vi "麦格纳通讯test.vi"() -> ()   [LabVIEW 2014]
panel:
  out "写入成功 7":bool
  out "读取成功 14":bool
  out "写入成功 6":bool
  out "读取成功 13":bool
  out "写入成功 5":bool
  out "读取成功 12":bool
  out "写入成功 4":bool
  out "读取成功 11":bool
  out "写入成功 3":bool
  out "读取成功 10":bool
  out "写入成功 2":bool
  out "读取成功 9":bool
  out "读取成功 8":bool
  out "读取成功 7":bool
  out "读取成功 6":bool
  out "读取成功 5":bool
  out "读取成功 4":bool
  out "读取成功 3":bool
  out "读取成功 2":bool
  out "写入成功":bool
  out "读取成功":bool
  out "ST150 write":u32
  out "ST150 read":u32[](array[numeric])
  out "ST150":bool
  out "ST130 write":u32
  out "ST130 read":u32[](array[numeric])
  out "ST130":bool
  out "ST140 write":u32
  out "ST140 read":u32[](array[numeric])
  out "ST140":bool
  out "ST70 write":u32
  out "ST70 read":u32[](array[numeric])
  out "ST70":bool
  out "ST80 write":u32
  out "ST80 read":u32[](array[numeric])
  out "ST80":bool
  out "ST90 write":u32
  out "ST90 read":u32[](array[numeric])
  out "ST90":bool
  out "ST100 write":u32
  out "ST100 read":u32[](array[numeric])
  out "ST100":bool
  out "ST110 write":u32
  out "ST110 read":u32[](array[numeric])
  out "ST110":bool
  out "ST120 write":u32
  out "ST120 read":u32[](array[numeric])
  out "ST120":bool
  out "ST60 write":u32
  out "ST50 write":u32
  out "ST40 write":u32
  out "ST30 write":u32
  out "ST20 write":u32
  out "ST60 read":u32[](array[numeric])
  out "ST50 read":u32[](array[numeric])
  out "ST40 read":u32[](array[numeric])
  out "ST30 read":u32[](array[numeric])
  out "ST20 read":u32[](array[numeric])
  out "ST10 write":u32
  out "ST10 read":u32[](array[numeric])
  out "ST60":bool
  out "ST50":bool
  out "ST40":bool
  out "ST30":bool
  out "ST20":bool
  out "ST10":bool
  in  "停止":bool
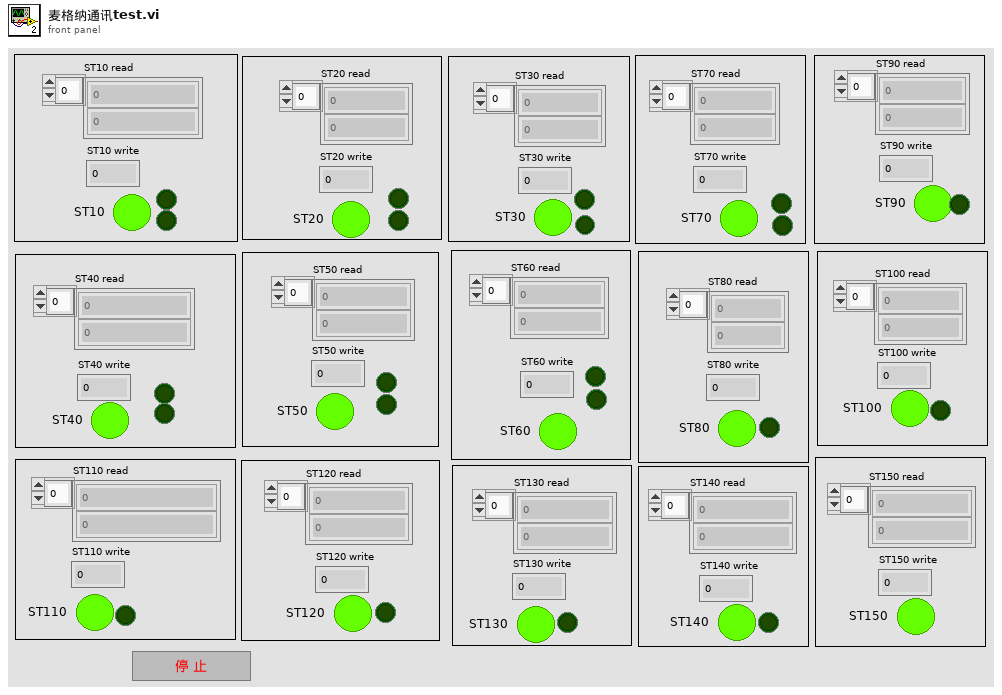
[diagram p1: front panel]
types:
  T1 = typedef "状态1.ctl" = enum16{"PLC通讯初始化", "读IO", "读DM", "写IO", "写DM", "-------------------", "仪表盘通讯初始化", "读数据", "保存曲线", "------------------", "错误"}
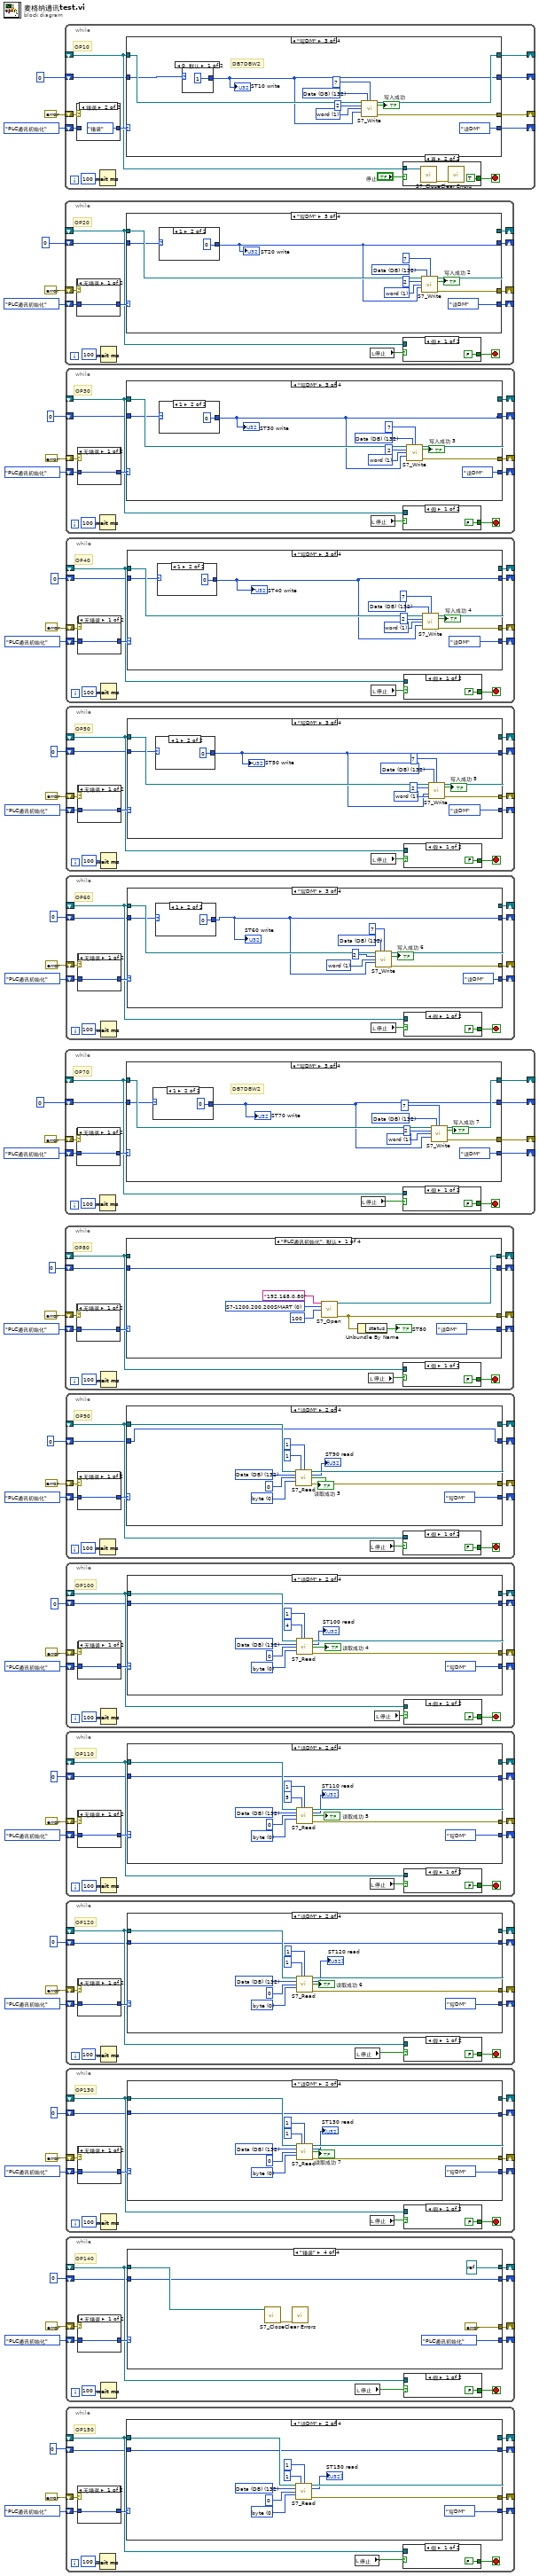
[diagram p0: block diagram]
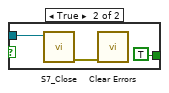
[diagram p2: hidden frame]
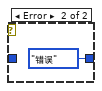
[diagram p3: hidden frame]
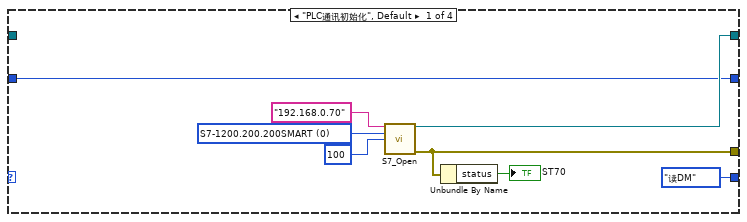
[diagram p4: hidden frame]
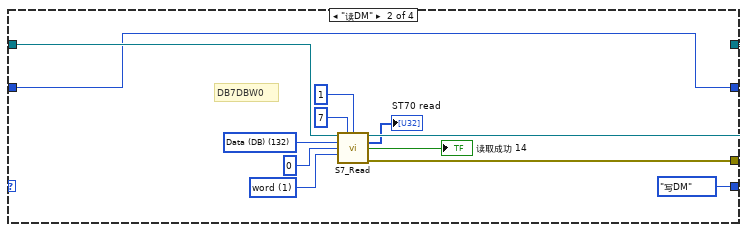
[diagram p5: hidden frame]
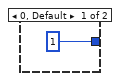
[diagram p6: hidden frame]
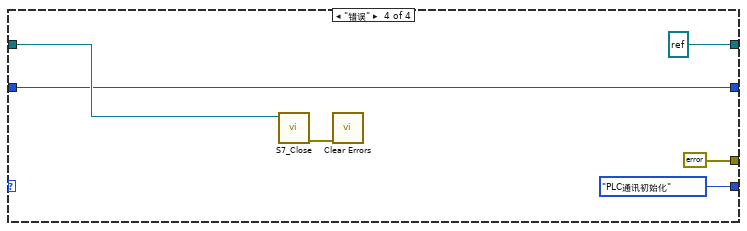
[diagram p7: hidden frame]
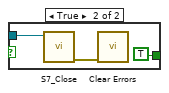
[diagram p8: hidden frame]
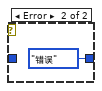
[diagram p9: hidden frame]
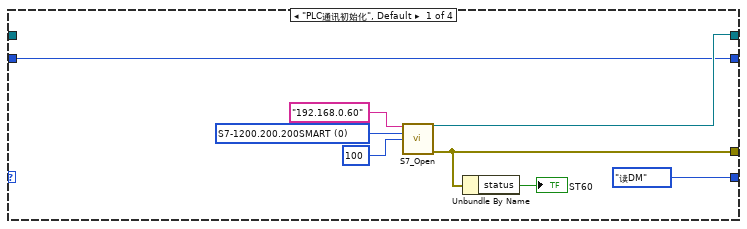
[diagram p10: hidden frame]
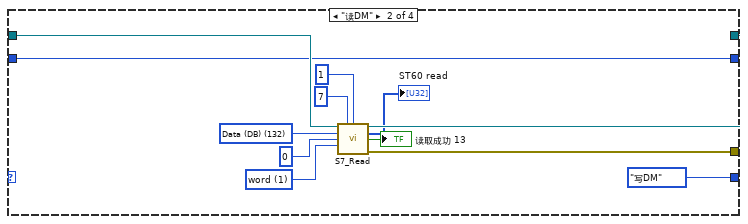
[diagram p11: hidden frame]
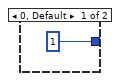
[diagram p12: hidden frame]
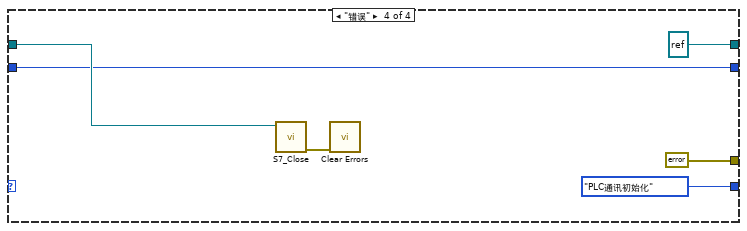
[diagram p13: hidden frame]
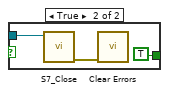
[diagram p14: hidden frame]
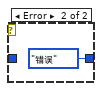
[diagram p15: hidden frame]
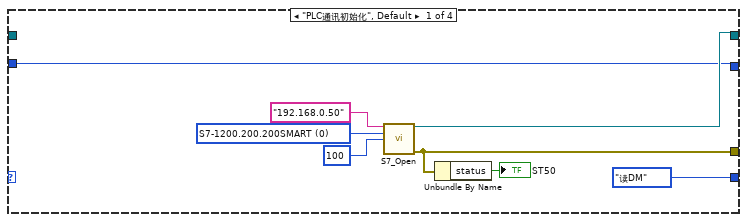
[diagram p16: hidden frame]
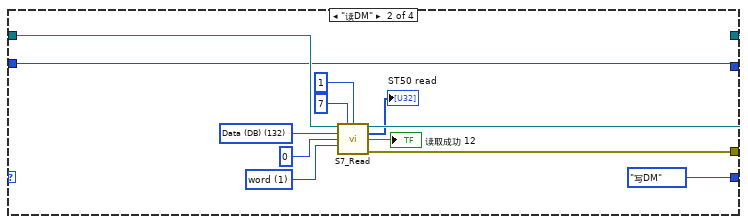
[diagram p17: hidden frame]
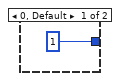
[diagram p18: hidden frame]
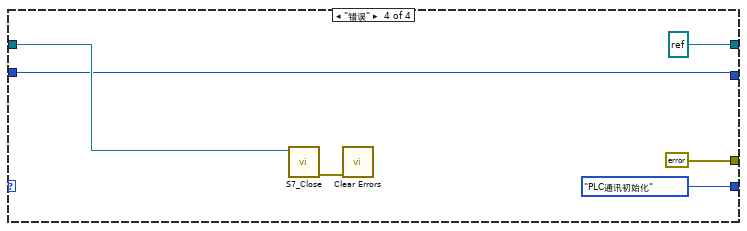
[diagram p19: hidden frame]
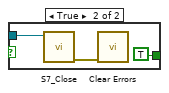
[diagram p20: hidden frame]
diagram:
  n1 = while {
    shift-right: [w51] -> _
    shift-left: 状态1."PLC通讯初始化" ("PLC状态") -> [w56]
    shift-right: [w53] -> _
    shift-left: errorcluster {"status"=FALSE, "code"=0, "source"=""} ("错误常量") -> [w57]
    shift-right: [w54] -> _
    shift-left: _ -> [w49]
    shift-right: [w46] -> _
    shift-left: u32 0 ("写入数据") -> [w47]
    stop <- w48 stop-if-true
    # "OP10"
    n2 = case shown="错误" w57 {
      tunnel: w56 -> [w62 _]
      tunnel: [w62 状态1."错误" ("PLC状态")] -> w55
      frame No Error {
      }
      frame Error {
      }
    }
    n3 = Wait (ms)(milliseconds to wait=u32 100 ("等待时间（毫秒）")) -> ()  [unwired: 1 out]
    n4 = case shown="\"写DM\"" w55 {
      tunnel: [w68 w78 w91 refnum<k5> refnum ("TCP")] -> w54
      tunnel: [w65 w77 w93 errorcluster {"status"=FALSE, "code"=0, "source"=""} ("error out")] -> w53
      tunnel: w49 -> [_ w79 w94 w102]
      tunnel: [状态1."读DM" ("PLC状态") 状态1."写DM" ("PLC状态") 状态1."读DM" ("PLC状态") 状态1."PLC通讯初始化" ("PLC状态")] -> w51
      tunnel: w47 -> [w66 w73 w86 w97]
      tunnel: [w66 w73 w85 w97] -> w46
      frame "PLC通讯初始化", Default {
        w70 = u8 0 items=["S7-1200.200.200SMART"=0, "S7-300"=2, "S7-400"=3] ("PLC 系列")
        n5 = call "S7_Open.vi"("IP 地址"="192.168.0.10", "PLC 系列"=w70, "超时（MS）"=100) -> ("TCP"=w68:refnum<k5>, "error out"=w65:errorcluster)  [unwired: 10 in, 1 out]
        n6 = Unbundle By Name(w65) -> ("status"=→"ST10":bool)
      }
      frame "读DM" {
        w80 = u16 1 items=["byte", "word", "Dword"] ("数据类型")
        w82 = u8 132 items=["I/O (P)"=128, "Input (I)"=129, "Output (Q)"=130, "Bit Memory (M)"=131, "Data (DB)"=132, "Instance Data (DI)"=133, "Local Data (L)"=134, "Predecessor Local Data (VL)"=135] ("寄存器类型")
        # "DB7DBW0"
        n7 = call "S7_Read.vi"("TCP"=w79, "DB #"=u16 7, "读取长度"=u16 1, "寄存器类型"=w82, "起始地址"=u32 0, "数据类型"=w80) -> ("TCP"=w78:refnum<k5>, "数据"=→"ST10 read":u32[], "读取成功"=→"读取成功":bool, "error out"=w77:errorcluster)  [unwired: 6 in]
      }
      frame "写DM" {
        w87 = u8 132 items=["I/O (P)"=128, "Input (I)"=129, "Output (Q)"=130, "Bit Memory (M)"=131, "Data (DB)"=132, "Instance Data (DI)"=133, "Local Data (L)"=134, "Predecessor Local Data (VL)"=135] ("寄存器类型")
        w89 = u16 1 items=["byte", "word", "Dword"] ("数据类型")
        # "DB7DBW2"
        n8 = case shown="0, 默认" w86 {
          tunnel: [u32 1 ("写入数据") u32 0 ("写入数据")] -> w85
          frame 0, Default {
          }
          frame 1 {
          }
        }
        "ST10 write" <- w85
        n9 = call "S7_Write.vi"("TCP"=w94, "寄存器类型"=w87, "DB #"=u16 7, "写入地址"=u32 2, "数据类型"=w89, "写入数据"=w85) -> ("TCP"=w91:refnum<k5>, "写入成功"=→"写入成功":bool, "error out"=w93:errorcluster)  [unwired: 7 in]
      }
      frame "错误" {
        n10 = call "S7_Close.vi"("TCP Connection Ref"=w102) -> ("error out"=w101:errorcluster)  [unwired: 10 in]
        n11 = call <vilib>:"Clear Errors.vi"("error in (no error)"=w101) -> ()  [unwired: 5 in, 2 out]
      }
    }
    n12 = case shown="真" "停止" {
      tunnel: w49 -> [_ w60]
      tunnel: [FALSE TRUE] -> w48
      frame False {
      }
      frame True {
        n13 = call "S7_Close.vi"("TCP Connection Ref"=w60) -> ("error out"=w61:errorcluster)  [unwired: 10 in]
        n14 = call <vilib>:"Clear Errors.vi"("error in (no error)"=w61) -> ()  [unwired: 5 in, 2 out]
      }
    }
  }
  n15 = while {
    shift-right: [w108] -> _
    shift-left: 状态1."PLC通讯初始化" ("PLC状态") -> [w113]
    shift-right: [w110] -> _
    shift-left: errorcluster {"status"=FALSE, "code"=0, "source"=""} ("错误常量") -> [w114]
    shift-right: [w111] -> _
    shift-left: _ -> [w107]
    shift-right: [w103] -> _
    shift-left: u32 0 ("写入数据") -> [w104]
    stop <- w106 stop-if-true
    # "OP20"
    n16 = case shown="无错误" w114 {
      tunnel: w113 -> [w119 _]
      tunnel: [w119 状态1."错误" ("PLC状态")] -> w112
      frame No Error {
      }
      frame Error {
      }
    }
    n17 = Wait (ms)(milliseconds to wait=u32 100 ("等待时间（毫秒）")) -> ()  [unwired: 1 out]
    n18 = case shown="\"写DM\"" w112 {
      tunnel: [w125 w135 w150 refnum<k5> refnum ("TCP")] -> w111
      tunnel: [w123 w134 w149 errorcluster {"status"=FALSE, "code"=0, "source"=""} ("error out")] -> w110
      tunnel: w107 -> [_ w136 w151 w159]
      tunnel: [状态1."读DM" ("PLC状态") 状态1."写DM" ("PLC状态") 状态1."读DM" ("PLC状态") 状态1."PLC通讯初始化" ("PLC状态")] -> w108
      tunnel: w104 -> [w121 w130 w143 w154]
      tunnel: [w121 w130 w142 w154] -> w103
      frame "PLC通讯初始化", Default {
        w127 = u8 0 items=["S7-1200.200.200SMART"=0, "S7-300"=2, "S7-400"=3] ("PLC 系列")
        n19 = call "S7_Open.vi"("IP 地址"="192.168.0.20", "PLC 系列"=w127, "超时（MS）"=100) -> ("TCP"=w125:refnum<k5>, "error out"=w123:errorcluster)  [unwired: 10 in, 1 out]
        n20 = Unbundle By Name(w123) -> ("status"=→"ST20":bool)
      }
      frame "读DM" {
        w137 = u16 1 items=["byte", "word", "Dword"] ("数据类型")
        w139 = u8 132 items=["I/O (P)"=128, "Input (I)"=129, "Output (Q)"=130, "Bit Memory (M)"=131, "Data (DB)"=132, "Instance Data (DI)"=133, "Local Data (L)"=134, "Predecessor Local Data (VL)"=135] ("寄存器类型")
        n21 = call "S7_Read.vi"("TCP"=w136, "DB #"=u16 7, "读取长度"=u16 1, "寄存器类型"=w139, "起始地址"=u32 0, "数据类型"=w137) -> ("TCP"=w135:refnum<k5>, "数据"=→"ST20 read":u32[], "读取成功"=→"读取成功 9":bool, "error out"=w134:errorcluster)  [unwired: 6 in]
      }
      frame "写DM" {
        w144 = u16 1 items=["byte", "word", "Dword"] ("数据类型")
        w146 = u8 132 items=["I/O (P)"=128, "Input (I)"=129, "Output (Q)"=130, "Bit Memory (M)"=131, "Data (DB)"=132, "Instance Data (DI)"=133, "Local Data (L)"=134, "Predecessor Local Data (VL)"=135] ("寄存器类型")
        n22 = case shown="1" w143 {
          tunnel: [u32 1 ("写入数据") u32 0 ("写入数据")] -> w142
          frame 0, Default {
          }
          frame 1 {
          }
        }
        "ST20 write" <- w142
        n23 = call "S7_Write.vi"("TCP"=w151, "寄存器类型"=w146, "DB #"=u16 7, "写入地址"=u32 2, "数据类型"=w144, "写入数据"=w142) -> ("TCP"=w150:refnum<k5>, "写入成功"=→"写入成功 2":bool, "error out"=w149:errorcluster)  [unwired: 7 in]
      }
      frame "错误" {
        n24 = call "S7_Close.vi"("TCP Connection Ref"=w159) -> ("error out"=w158:errorcluster)  [unwired: 10 in]
        n25 = call <vilib>:"Clear Errors.vi"("error in (no error)"=w158) -> ()  [unwired: 5 in, 2 out]
      }
    }
    n26 = local read "停止"() -> (w105:bool)
    n27 = case shown="假" w105 {
      tunnel: w107 -> [_ w117]
      tunnel: [FALSE TRUE] -> w106
      frame False {
      }
      frame True {
        n28 = call "S7_Close.vi"("TCP Connection Ref"=w117) -> ("error out"=w118:errorcluster)  [unwired: 10 in]
        n29 = call <vilib>:"Clear Errors.vi"("error in (no error)"=w118) -> ()  [unwired: 5 in, 2 out]
      }
    }
  }
  n30 = while {
    shift-right: [w165] -> _
    shift-left: 状态1."PLC通讯初始化" ("PLC状态") -> [w170]
    shift-right: [w167] -> _
    shift-left: errorcluster {"status"=FALSE, "code"=0, "source"=""} ("错误常量") -> [w171]
    shift-right: [w168] -> _
    shift-left: _ -> [w164]
    shift-right: [w161] -> _
    shift-left: u32 0 ("写入数据") -> [w162]
    stop <- w163 stop-if-true
    # "OP70"
    n31 = case shown="无错误" w171 {
      tunnel: w170 -> [w176 _]
      tunnel: [w176 状态1."错误" ("PLC状态")] -> w169
      frame No Error {
      }
      frame Error {
      }
    }
    n32 = Wait (ms)(milliseconds to wait=u32 100 ("等待时间（毫秒）")) -> ()  [unwired: 1 out]
    n33 = case shown="\"写DM\"" w169 {
      tunnel: [w182 w192 w205 refnum<k5> refnum ("TCP")] -> w168
      tunnel: [w180 w191 w207 errorcluster {"status"=FALSE, "code"=0, "source"=""} ("error out")] -> w167
      tunnel: w164 -> [_ w193 w208 w216]
      tunnel: [状态1."读DM" ("PLC状态") 状态1."写DM" ("PLC状态") 状态1."读DM" ("PLC状态") 状态1."PLC通讯初始化" ("PLC状态")] -> w165
      tunnel: w162 -> [w178 w187 w200 w211]
      tunnel: [w178 w187 w199 w211] -> w161
      frame "PLC通讯初始化", Default {
        w184 = u8 0 items=["S7-1200.200.200SMART"=0, "S7-300"=2, "S7-400"=3] ("PLC 系列")
        n34 = call "S7_Open.vi"("IP 地址"="192.168.0.70", "PLC 系列"=w184, "超时（MS）"=100) -> ("TCP"=w182:refnum<k5>, "error out"=w180:errorcluster)  [unwired: 10 in, 1 out]
        n35 = Unbundle By Name(w180) -> ("status"=→"ST70":bool)
      }
      frame "读DM" {
        w194 = u16 1 items=["byte", "word", "Dword"] ("数据类型")
        w196 = u8 132 items=["I/O (P)"=128, "Input (I)"=129, "Output (Q)"=130, "Bit Memory (M)"=131, "Data (DB)"=132, "Instance Data (DI)"=133, "Local Data (L)"=134, "Predecessor Local Data (VL)"=135] ("寄存器类型")
        # "DB7DBW0"
        n36 = call "S7_Read.vi"("TCP"=w193, "DB #"=u16 7, "读取长度"=u16 1, "寄存器类型"=w196, "起始地址"=u32 0, "数据类型"=w194) -> ("TCP"=w192:refnum<k5>, "数据"=→"ST70 read":u32[], "读取成功"=→"读取成功 14":bool, "error out"=w191:errorcluster)  [unwired: 6 in]
      }
      frame "写DM" {
        w201 = u8 132 items=["I/O (P)"=128, "Input (I)"=129, "Output (Q)"=130, "Bit Memory (M)"=131, "Data (DB)"=132, "Instance Data (DI)"=133, "Local Data (L)"=134, "Predecessor Local Data (VL)"=135] ("寄存器类型")
        w203 = u16 1 items=["byte", "word", "Dword"] ("数据类型")
        # "DB7DBW2"
        n37 = case shown="1" w200 {
          tunnel: [u32 1 ("写入数据") u32 0 ("写入数据")] -> w199
          frame 0, Default {
          }
          frame 1 {
          }
        }
        "ST70 write" <- w199
        n38 = call "S7_Write.vi"("TCP"=w208, "寄存器类型"=w201, "DB #"=u16 7, "写入地址"=u32 2, "数据类型"=w203, "写入数据"=w199) -> ("TCP"=w205:refnum<k5>, "写入成功"=→"写入成功 7":bool, "error out"=w207:errorcluster)  [unwired: 7 in]
      }
      frame "错误" {
        n39 = call "S7_Close.vi"("TCP Connection Ref"=w216) -> ("error out"=w215:errorcluster)  [unwired: 10 in]
        n40 = call <vilib>:"Clear Errors.vi"("error in (no error)"=w215) -> ()  [unwired: 5 in, 2 out]
      }
    }
    n41 = local read "停止"() -> (w160:bool)
    n42 = case shown="假" w160 {
      tunnel: w164 -> [_ w174]
      tunnel: [FALSE TRUE] -> w163
      frame False {
      }
      frame True {
        n43 = call "S7_Close.vi"("TCP Connection Ref"=w174) -> ("error out"=w175:errorcluster)  [unwired: 10 in]
        n44 = call <vilib>:"Clear Errors.vi"("error in (no error)"=w175) -> ()  [unwired: 5 in, 2 out]
      }
    }
  }
  n45 = while {
    shift-right: [w222] -> _
    shift-left: 状态1."PLC通讯初始化" ("PLC状态") -> [w227]
    shift-right: [w224] -> _
    shift-left: errorcluster {"status"=FALSE, "code"=0, "source"=""} ("错误常量") -> [w228]
    shift-right: [w225] -> _
    shift-left: _ -> [w221]
    shift-right: [w218] -> _
    shift-left: u32 0 ("写入数据") -> [w219]
    stop <- w220 stop-if-true
    # "OP80"
    n46 = case shown="无错误" w228 {
      tunnel: w227 -> [w233 _]
      tunnel: [w233 状态1."错误" ("PLC状态")] -> w226
      frame No Error {
      }
      frame Error {
      }
    }
    n47 = Wait (ms)(milliseconds to wait=u32 100 ("等待时间（毫秒）")) -> ()  [unwired: 1 out]
    n48 = case shown="\"PLC通讯初始化\", 默认" w226 {
      tunnel: [w239 w249 w259 refnum<k5> refnum ("TCP")] -> w225
      tunnel: [w237 w248 w258 errorcluster {"status"=FALSE, "code"=0, "source"=""} ("error out")] -> w224
      tunnel: w221 -> [_ w250 w260 w280]
      tunnel: [状态1."读DM" ("PLC状态") 状态1."写DM" ("PLC状态") 状态1."读DM" ("PLC状态") 状态1."PLC通讯初始化" ("PLC状态")] -> w222
      tunnel: w219 -> [w235 w244 w256 w275]
      tunnel: [w235 w244 w255 w275] -> w218
      frame "PLC通讯初始化", Default {
        w241 = u8 0 items=["S7-1200.200.200SMART"=0, "S7-300"=2, "S7-400"=3] ("PLC 系列")
        n49 = call "S7_Open.vi"("IP 地址"="192.168.0.80", "PLC 系列"=w241, "超时（MS）"=100) -> ("TCP"=w239:refnum<k5>, "error out"=w237:errorcluster)  [unwired: 10 in, 1 out]
        n50 = Unbundle By Name(w237) -> ("status"=→"ST80":bool)
      }
      frame "读DM" {
        w251 = u16 0 items=["byte", "word", "Dword"] ("数据类型")
        w253 = u8 132 items=["I/O (P)"=128, "Input (I)"=129, "Output (Q)"=130, "Bit Memory (M)"=131, "Data (DB)"=132, "Instance Data (DI)"=133, "Local Data (L)"=134, "Predecessor Local Data (VL)"=135] ("寄存器类型")
        n51 = call "S7_Read.vi"("TCP"=w250, "DB #"=u16 8, "读取长度"=u16 1, "寄存器类型"=w253, "起始地址"=u32 0, "数据类型"=w251) -> ("TCP"=w249:refnum<k5>, "数据"=→"ST80 read":u32[], "读取成功"=→"读取成功 2":bool, "error out"=w248:errorcluster)  [unwired: 6 in]
      }
      frame "写DM" {
        n52 = disable-structure shown="启用" {
          disable-tunnel: w260 -> [w269 w274]
          disable-tunnel: [w268 w274] -> w259
          disable-tunnel: [w267 errorcluster {"status"=FALSE, "code"=0, "source"=""} ("error out")] -> w258
          disable-tunnel: w256 -> [w262 w273]
          disable-tunnel: [w261 w273] -> w255
          frame Disabled {
            w263 = u16 1 items=["byte", "word", "Dword"] ("数据类型")
            w265 = u8 132 items=["I/O (P)"=128, "Input (I)"=129, "Output (Q)"=130, "Bit Memory (M)"=131, "Data (DB)"=132, "Instance Data (DI)"=133, "Local Data (L)"=134, "Predecessor Local Data (VL)"=135] ("寄存器类型")
            n53 = case shown="1" w262 {
              tunnel: [u32 1 ("写入数据") u32 0 ("写入数据")] -> w261
              frame 0, Default {
              }
              frame 1 {
              }
            }
            "ST80 write" <- w261
            n54 = call "S7_Write.vi"("TCP"=w269, "寄存器类型"=w265, "DB #"=u16 7, "写入地址"=u32 2, "数据类型"=w263, "写入数据"=w261) -> ("TCP"=w268:refnum<k5>, "error out"=w267:errorcluster)  [unwired: 7 in, 1 out]
          }
          frame Enabled {
          }
        }
      }
      frame "错误" {
        n55 = call "S7_Close.vi"("TCP Connection Ref"=w280) -> ("error out"=w279:errorcluster)  [unwired: 10 in]
        n56 = call <vilib>:"Clear Errors.vi"("error in (no error)"=w279) -> ()  [unwired: 5 in, 2 out]
      }
    }
    n57 = local read "停止"() -> (w217:bool)
    n58 = case shown="假" w217 {
      tunnel: w221 -> [_ w231]
      tunnel: [FALSE TRUE] -> w220
      frame False {
      }
      frame True {
        n59 = call "S7_Close.vi"("TCP Connection Ref"=w231) -> ("error out"=w232:errorcluster)  [unwired: 10 in]
        n60 = call <vilib>:"Clear Errors.vi"("error in (no error)"=w232) -> ()  [unwired: 5 in, 2 out]
      }
    }
  }
  n61 = while {
    shift-right: [w286] -> _
    shift-left: 状态1."PLC通讯初始化" ("PLC状态") -> [w291]
    shift-right: [w288] -> _
    shift-left: errorcluster {"status"=FALSE, "code"=0, "source"=""} ("错误常量") -> [w292]
    shift-right: [w289] -> _
    shift-left: _ -> [w285]
    shift-right: [w281] -> _
    shift-left: u32 0 ("写入数据") -> [w282]
    stop <- w284 stop-if-true
    # "OP30"
    n62 = case shown="无错误" w292 {
      tunnel: w291 -> [w297 _]
      tunnel: [w297 状态1."错误" ("PLC状态")] -> w290
      frame No Error {
      }
      frame Error {
      }
    }
    n63 = Wait (ms)(milliseconds to wait=u32 100 ("等待时间（毫秒）")) -> ()  [unwired: 1 out]
    n64 = case shown="\"写DM\"" w290 {
      tunnel: [w303 w313 w328 refnum<k5> refnum ("TCP")] -> w289
      tunnel: [w300 w312 w327 errorcluster {"status"=FALSE, "code"=0, "source"=""} ("error out")] -> w288
      tunnel: w285 -> [_ w314 w329 w337]
      tunnel: [状态1."读DM" ("PLC状态") 状态1."写DM" ("PLC状态") 状态1."读DM" ("PLC状态") 状态1."PLC通讯初始化" ("PLC状态")] -> w286
      tunnel: w282 -> [w299 w308 w325 w332]
      tunnel: [w299 w308 w320 w332] -> w281
      frame "PLC通讯初始化", Default {
        w305 = u8 0 items=["S7-1200.200.200SMART"=0, "S7-300"=2, "S7-400"=3] ("PLC 系列")
        n65 = call "S7_Open.vi"("IP 地址"="192.168.0.30", "PLC 系列"=w305, "超时（MS）"=100) -> ("TCP"=w303:refnum<k5>, "error out"=w300:errorcluster)  [unwired: 10 in, 1 out]
        n66 = Unbundle By Name(w300) -> ("status"=→"ST30":bool)
      }
      frame "读DM" {
        w315 = u16 1 items=["byte", "word", "Dword"] ("数据类型")
        w317 = u8 132 items=["I/O (P)"=128, "Input (I)"=129, "Output (Q)"=130, "Bit Memory (M)"=131, "Data (DB)"=132, "Instance Data (DI)"=133, "Local Data (L)"=134, "Predecessor Local Data (VL)"=135] ("寄存器类型")
        n67 = call "S7_Read.vi"("TCP"=w314, "DB #"=u16 7, "读取长度"=u16 1, "寄存器类型"=w317, "起始地址"=u32 0, "数据类型"=w315) -> ("TCP"=w313:refnum<k5>, "数据"=→"ST30 read":u32[], "读取成功"=→"读取成功 10":bool, "error out"=w312:errorcluster)  [unwired: 6 in]
      }
      frame "写DM" {
        w321 = u16 1 items=["byte", "word", "Dword"] ("数据类型")
        w324 = u8 132 items=["I/O (P)"=128, "Input (I)"=129, "Output (Q)"=130, "Bit Memory (M)"=131, "Data (DB)"=132, "Instance Data (DI)"=133, "Local Data (L)"=134, "Predecessor Local Data (VL)"=135] ("寄存器类型")
        n68 = case shown="1" w325 {
          tunnel: [u32 1 ("写入数据") u32 0 ("写入数据")] -> w320
          frame 0, Default {
          }
          frame 1 {
          }
        }
        "ST30 write" <- w320
        n69 = call "S7_Write.vi"("TCP"=w329, "寄存器类型"=w324, "DB #"=u16 7, "写入地址"=u32 2, "数据类型"=w321, "写入数据"=w320) -> ("TCP"=w328:refnum<k5>, "写入成功"=→"写入成功 3":bool, "error out"=w327:errorcluster)  [unwired: 7 in]
      }
      frame "错误" {
        n70 = call "S7_Close.vi"("TCP Connection Ref"=w337) -> ("error out"=w336:errorcluster)  [unwired: 10 in]
        n71 = call <vilib>:"Clear Errors.vi"("error in (no error)"=w336) -> ()  [unwired: 5 in, 2 out]
      }
    }
    n72 = local read "停止"() -> (w283:bool)
    n73 = case shown="假" w283 {
      tunnel: w285 -> [_ w295]
      tunnel: [FALSE TRUE] -> w284
      frame False {
      }
      frame True {
        n74 = call "S7_Close.vi"("TCP Connection Ref"=w295) -> ("error out"=w296:errorcluster)  [unwired: 10 in]
        n75 = call <vilib>:"Clear Errors.vi"("error in (no error)"=w296) -> ()  [unwired: 5 in, 2 out]
      }
    }
  }
  n76 = while {
    shift-right: [w343] -> _
    shift-left: 状态1."PLC通讯初始化" ("PLC状态") -> [w348]
    shift-right: [w345] -> _
    shift-left: errorcluster {"status"=FALSE, "code"=0, "source"=""} ("错误常量") -> [w349]
    shift-right: [w346] -> _
    shift-left: _ -> [w342]
    shift-right: [w339] -> _
    shift-left: u32 0 ("写入数据") -> [w340]
    stop <- w341 stop-if-true
    # "OP90"
    n77 = case shown="无错误" w349 {
      tunnel: w348 -> [w354 _]
      tunnel: [w354 状态1."错误" ("PLC状态")] -> w347
      frame No Error {
      }
      frame Error {
      }
    }
    n78 = Wait (ms)(milliseconds to wait=u32 100 ("等待时间（毫秒）")) -> ()  [unwired: 1 out]
    n79 = case shown="\"读DM\"" w347 {
      tunnel: [w360 w370 w380 refnum<k5> refnum ("TCP")] -> w346
      tunnel: [w357 w369 w379 errorcluster {"status"=FALSE, "code"=0, "source"=""} ("error out")] -> w345
      tunnel: w342 -> [_ w371 w381 w401]
      tunnel: [状态1."读DM" ("PLC状态") 状态1."写DM" ("PLC状态") 状态1."读DM" ("PLC状态") 状态1."PLC通讯初始化" ("PLC状态")] -> w343
      tunnel: w340 -> [w356 w365 w377 w396]
      tunnel: [w356 w365 w376 w396] -> w339
      frame "PLC通讯初始化", Default {
        w362 = u8 0 items=["S7-1200.200.200SMART"=0, "S7-300"=2, "S7-400"=3] ("PLC 系列")
        n80 = call "S7_Open.vi"("IP 地址"="192.168.0.90", "PLC 系列"=w362, "超时（MS）"=100) -> ("TCP"=w360:refnum<k5>, "error out"=w357:errorcluster)  [unwired: 10 in, 1 out]
        n81 = Unbundle By Name(w357) -> ("status"=→"ST90":bool)
      }
      frame "读DM" {
        w372 = u16 0 items=["byte", "word", "Dword"] ("数据类型")
        w374 = u8 132 items=["I/O (P)"=128, "Input (I)"=129, "Output (Q)"=130, "Bit Memory (M)"=131, "Data (DB)"=132, "Instance Data (DI)"=133, "Local Data (L)"=134, "Predecessor Local Data (VL)"=135] ("寄存器类型")
        n82 = call "S7_Read.vi"("TCP"=w371, "DB #"=u16 1, "读取长度"=u16 1, "寄存器类型"=w374, "起始地址"=u32 0, "数据类型"=w372) -> ("TCP"=w370:refnum<k5>, "数据"=→"ST90 read":u32[], "读取成功"=→"读取成功 3":bool, "error out"=w369:errorcluster)  [unwired: 6 in]
      }
      frame "写DM" {
        n83 = disable-structure shown="启用" {
          disable-tunnel: w381 -> [w390 w394]
          disable-tunnel: [w389 w394] -> w380
          disable-tunnel: [w388 errorcluster {"status"=FALSE, "code"=0, "source"=""} ("error out")] -> w379
          disable-tunnel: w377 -> [w387 w395]
          disable-tunnel: [w382 w395] -> w376
          frame Disabled {
            w383 = u16 1 items=["byte", "word", "Dword"] ("数据类型")
            w386 = u8 132 items=["I/O (P)"=128, "Input (I)"=129, "Output (Q)"=130, "Bit Memory (M)"=131, "Data (DB)"=132, "Instance Data (DI)"=133, "Local Data (L)"=134, "Predecessor Local Data (VL)"=135] ("寄存器类型")
            n84 = case shown="1" w387 {
              tunnel: [u32 1 ("写入数据") u32 0 ("写入数据")] -> w382
              frame 0, Default {
              }
              frame 1 {
              }
            }
            "ST90 write" <- w382
            n85 = call "S7_Write.vi"("TCP"=w390, "寄存器类型"=w386, "DB #"=u16 7, "写入地址"=u32 2, "数据类型"=w383, "写入数据"=w382) -> ("TCP"=w389:refnum<k5>, "error out"=w388:errorcluster)  [unwired: 7 in, 1 out]
          }
          frame Enabled {
          }
        }
      }
      frame "错误" {
        n86 = call "S7_Close.vi"("TCP Connection Ref"=w401) -> ("error out"=w400:errorcluster)  [unwired: 10 in]
        n87 = call <vilib>:"Clear Errors.vi"("error in (no error)"=w400) -> ()  [unwired: 5 in, 2 out]
      }
    }
    n88 = local read "停止"() -> (w338:bool)
    n89 = case shown="假" w338 {
      tunnel: w342 -> [_ w352]
      tunnel: [FALSE TRUE] -> w341
      frame False {
      }
      frame True {
        n90 = call "S7_Close.vi"("TCP Connection Ref"=w352) -> ("error out"=w353:errorcluster)  [unwired: 10 in]
        n91 = call <vilib>:"Clear Errors.vi"("error in (no error)"=w353) -> ()  [unwired: 5 in, 2 out]
      }
    }
  }
  n92 = while {
    shift-right: [w407] -> _
    shift-left: 状态1."PLC通讯初始化" ("PLC状态") -> [w412]
    shift-right: [w409] -> _
    shift-left: errorcluster {"status"=FALSE, "code"=0, "source"=""} ("错误常量") -> [w413]
    shift-right: [w410] -> _
    shift-left: _ -> [w406]
    shift-right: [w403] -> _
    shift-left: u32 0 ("写入数据") -> [w404]
    stop <- w405 stop-if-true
    # "OP150"
    n93 = case shown="无错误" w413 {
      tunnel: w412 -> [w418 _]
      tunnel: [w418 状态1."错误" ("PLC状态")] -> w411
      frame No Error {
      }
      frame Error {
      }
    }
    n94 = Wait (ms)(milliseconds to wait=u32 100 ("等待时间（毫秒）")) -> ()  [unwired: 1 out]
    n95 = case shown="\"读DM\"" w411 {
      tunnel: [w424 w433 w443 refnum<k5> refnum ("TCP")] -> w410
      tunnel: [w421 w432 w442 errorcluster {"status"=FALSE, "code"=0, "source"=""} ("error out")] -> w409
      tunnel: w406 -> [_ w434 w444 w464]
      tunnel: [状态1."读DM" ("PLC状态") 状态1."写DM" ("PLC状态") 状态1."读DM" ("PLC状态") 状态1."PLC通讯初始化" ("PLC状态")] -> w407
      tunnel: w404 -> [w420 w428 w440 w459]
      tunnel: [w420 w428 w439 w459] -> w403
      frame "PLC通讯初始化", Default {
        w426 = u8 0 items=["S7-1200.200.200SMART"=0, "S7-300"=2, "S7-400"=3] ("PLC 系列")
        n96 = call "S7_Open.vi"("IP 地址"="192.168.0.150", "PLC 系列"=w426, "超时（MS）"=100) -> ("TCP"=w424:refnum<k5>, "error out"=w421:errorcluster)  [unwired: 10 in, 1 out]
        n97 = Unbundle By Name(w421) -> ("status"=→"ST150":bool)
      }
      frame "读DM" {
        w435 = u16 0 items=["byte", "word", "Dword"] ("数据类型")
        w437 = u8 132 items=["I/O (P)"=128, "Input (I)"=129, "Output (Q)"=130, "Bit Memory (M)"=131, "Data (DB)"=132, "Instance Data (DI)"=133, "Local Data (L)"=134, "Predecessor Local Data (VL)"=135] ("寄存器类型")
        n98 = call "S7_Read.vi"("TCP"=w434, "DB #"=u16 1, "读取长度"=u16 1, "寄存器类型"=w437, "起始地址"=u32 0, "数据类型"=w435) -> ("TCP"=w433:refnum<k5>, "数据"=→"ST150 read":u32[], "error out"=w432:errorcluster)  [unwired: 6 in, 1 out]
      }
      frame "写DM" {
        n99 = disable-structure shown="启用" {
          disable-tunnel: w444 -> [w453 w457]
          disable-tunnel: [w452 w457] -> w443
          disable-tunnel: [w451 errorcluster {"status"=FALSE, "code"=0, "source"=""} ("error out")] -> w442
          disable-tunnel: w440 -> [w450 w458]
          disable-tunnel: [w445 w458] -> w439
          frame Disabled {
            w446 = u16 1 items=["byte", "word", "Dword"] ("数据类型")
            w448 = u8 132 items=["I/O (P)"=128, "Input (I)"=129, "Output (Q)"=130, "Bit Memory (M)"=131, "Data (DB)"=132, "Instance Data (DI)"=133, "Local Data (L)"=134, "Predecessor Local Data (VL)"=135] ("寄存器类型")
            n100 = case shown="1" w450 {
              tunnel: [u32 1 ("写入数据") u32 0 ("写入数据")] -> w445
              frame 0, Default {
              }
              frame 1 {
              }
            }
            "ST150 write" <- w445
            n101 = call "S7_Write.vi"("TCP"=w453, "寄存器类型"=w448, "DB #"=u16 7, "写入地址"=u32 2, "数据类型"=w446, "写入数据"=w445) -> ("TCP"=w452:refnum<k5>, "error out"=w451:errorcluster)  [unwired: 7 in, 1 out]
          }
          frame Enabled {
          }
        }
      }
      frame "错误" {
        n102 = call "S7_Close.vi"("TCP Connection Ref"=w464) -> ("error out"=w463:errorcluster)  [unwired: 10 in]
        n103 = call <vilib>:"Clear Errors.vi"("error in (no error)"=w463) -> ()  [unwired: 5 in, 2 out]
      }
    }
    n104 = local read "停止"() -> (w402:bool)
    n105 = case shown="假" w402 {
      tunnel: w406 -> [_ w416]
      tunnel: [FALSE TRUE] -> w405
      frame False {
      }
      frame True {
        n106 = call "S7_Close.vi"("TCP Connection Ref"=w416) -> ("error out"=w417:errorcluster)  [unwired: 10 in]
        n107 = call <vilib>:"Clear Errors.vi"("error in (no error)"=w417) -> ()  [unwired: 5 in, 2 out]
      }
    }
  }
  n108 = while {
    shift-right: [w470] -> _
    shift-left: 状态1."PLC通讯初始化" ("PLC状态") -> [w475]
    shift-right: [w472] -> _
    shift-left: errorcluster {"status"=FALSE, "code"=0, "source"=""} ("错误常量") -> [w476]
    shift-right: [w473] -> _
    shift-left: _ -> [w469]
    shift-right: [w465] -> _
    shift-left: u32 0 ("写入数据") -> [w466]
    stop <- w468 stop-if-true
    # "OP40"
    n109 = case shown="无错误" w476 {
      tunnel: w475 -> [w481 _]
      tunnel: [w481 状态1."错误" ("PLC状态")] -> w474
      frame No Error {
      }
      frame Error {
      }
    }
    n110 = Wait (ms)(milliseconds to wait=u32 100 ("等待时间（毫秒）")) -> ()  [unwired: 1 out]
    n111 = case shown="\"写DM\"" w474 {
      tunnel: [w487 w497 w512 refnum<k5> refnum ("TCP")] -> w473
      tunnel: [w484 w496 w511 errorcluster {"status"=FALSE, "code"=0, "source"=""} ("error out")] -> w472
      tunnel: w469 -> [_ w498 w513 w521]
      tunnel: [状态1."读DM" ("PLC状态") 状态1."写DM" ("PLC状态") 状态1."读DM" ("PLC状态") 状态1."PLC通讯初始化" ("PLC状态")] -> w470
      tunnel: w466 -> [w483 w492 w509 w516]
      tunnel: [w483 w492 w504 w516] -> w465
      frame "PLC通讯初始化", Default {
        w489 = u8 0 items=["S7-1200.200.200SMART"=0, "S7-300"=2, "S7-400"=3] ("PLC 系列")
        n112 = call "S7_Open.vi"("IP 地址"="192.168.0.40", "PLC 系列"=w489, "超时（MS）"=100) -> ("TCP"=w487:refnum<k5>, "error out"=w484:errorcluster)  [unwired: 10 in, 1 out]
        n113 = Unbundle By Name(w484) -> ("status"=→"ST40":bool)
      }
      frame "读DM" {
        w499 = u16 1 items=["byte", "word", "Dword"] ("数据类型")
        w501 = u8 132 items=["I/O (P)"=128, "Input (I)"=129, "Output (Q)"=130, "Bit Memory (M)"=131, "Data (DB)"=132, "Instance Data (DI)"=133, "Local Data (L)"=134, "Predecessor Local Data (VL)"=135] ("寄存器类型")
        n114 = call "S7_Read.vi"("TCP"=w498, "DB #"=u16 7, "读取长度"=u16 1, "寄存器类型"=w501, "起始地址"=u32 0, "数据类型"=w499) -> ("TCP"=w497:refnum<k5>, "数据"=→"ST40 read":u32[], "读取成功"=→"读取成功 11":bool, "error out"=w496:errorcluster)  [unwired: 6 in]
      }
      frame "写DM" {
        w505 = u16 1 items=["byte", "word", "Dword"] ("数据类型")
        w507 = u8 132 items=["I/O (P)"=128, "Input (I)"=129, "Output (Q)"=130, "Bit Memory (M)"=131, "Data (DB)"=132, "Instance Data (DI)"=133, "Local Data (L)"=134, "Predecessor Local Data (VL)"=135] ("寄存器类型")
        n115 = case shown="1" w509 {
          tunnel: [u32 1 ("写入数据") u32 0 ("写入数据")] -> w504
          frame 0, Default {
          }
          frame 1 {
          }
        }
        "ST40 write" <- w504
        n116 = call "S7_Write.vi"("TCP"=w513, "寄存器类型"=w507, "DB #"=u16 7, "写入地址"=u32 2, "数据类型"=w505, "写入数据"=w504) -> ("TCP"=w512:refnum<k5>, "写入成功"=→"写入成功 4":bool, "error out"=w511:errorcluster)  [unwired: 7 in]
      }
      frame "错误" {
        n117 = call "S7_Close.vi"("TCP Connection Ref"=w521) -> ("error out"=w520:errorcluster)  [unwired: 10 in]
        n118 = call <vilib>:"Clear Errors.vi"("error in (no error)"=w520) -> ()  [unwired: 5 in, 2 out]
      }
    }
    n119 = local read "停止"() -> (w467:bool)
    n120 = case shown="假" w467 {
      tunnel: w469 -> [_ w479]
      tunnel: [FALSE TRUE] -> w468
      frame False {
      }
      frame True {
        n121 = call "S7_Close.vi"("TCP Connection Ref"=w479) -> ("error out"=w480:errorcluster)  [unwired: 10 in]
        n122 = call <vilib>:"Clear Errors.vi"("error in (no error)"=w480) -> ()  [unwired: 5 in, 2 out]
      }
    }
  }
  n123 = while {
    shift-right: [w527] -> _
    shift-left: 状态1."PLC通讯初始化" ("PLC状态") -> [w532]
    shift-right: [w529] -> _
    shift-left: errorcluster {"status"=FALSE, "code"=0, "source"=""} ("错误常量") -> [w533]
    shift-right: [w530] -> _
    shift-left: _ -> [w526]
    shift-right: [w522] -> _
    shift-left: u32 0 ("写入数据") -> [w523]
    stop <- w525 stop-if-true
    # "OP50"
    n124 = case shown="无错误" w533 {
      tunnel: w532 -> [w538 _]
      tunnel: [w538 状态1."错误" ("PLC状态")] -> w531
      frame No Error {
      }
      frame Error {
      }
    }
    n125 = Wait (ms)(milliseconds to wait=u32 100 ("等待时间（毫秒）")) -> ()  [unwired: 1 out]
    n126 = case shown="\"写DM\"" w531 {
      tunnel: [w544 w554 w569 refnum<k5> refnum ("TCP")] -> w530
      tunnel: [w541 w553 w568 errorcluster {"status"=FALSE, "code"=0, "source"=""} ("error out")] -> w529
      tunnel: w526 -> [_ w555 w570 w578]
      tunnel: [状态1."读DM" ("PLC状态") 状态1."写DM" ("PLC状态") 状态1."读DM" ("PLC状态") 状态1."PLC通讯初始化" ("PLC状态")] -> w527
      tunnel: w523 -> [w540 w549 w566 w573]
      tunnel: [w540 w549 w561 w573] -> w522
      frame "PLC通讯初始化", Default {
        w546 = u8 0 items=["S7-1200.200.200SMART"=0, "S7-300"=2, "S7-400"=3] ("PLC 系列")
        n127 = call "S7_Open.vi"("IP 地址"="192.168.0.50", "PLC 系列"=w546, "超时（MS）"=100) -> ("TCP"=w544:refnum<k5>, "error out"=w541:errorcluster)  [unwired: 10 in, 1 out]
        n128 = Unbundle By Name(w541) -> ("status"=→"ST50":bool)
      }
      frame "读DM" {
        w556 = u16 1 items=["byte", "word", "Dword"] ("数据类型")
        w558 = u8 132 items=["I/O (P)"=128, "Input (I)"=129, "Output (Q)"=130, "Bit Memory (M)"=131, "Data (DB)"=132, "Instance Data (DI)"=133, "Local Data (L)"=134, "Predecessor Local Data (VL)"=135] ("寄存器类型")
        n129 = call "S7_Read.vi"("TCP"=w555, "DB #"=u16 7, "读取长度"=u16 1, "寄存器类型"=w558, "起始地址"=u32 0, "数据类型"=w556) -> ("TCP"=w554:refnum<k5>, "数据"=→"ST50 read":u32[], "读取成功"=→"读取成功 12":bool, "error out"=w553:errorcluster)  [unwired: 6 in]
      }
      frame "写DM" {
        w562 = u16 1 items=["byte", "word", "Dword"] ("数据类型")
        w564 = u8 132 items=["I/O (P)"=128, "Input (I)"=129, "Output (Q)"=130, "Bit Memory (M)"=131, "Data (DB)"=132, "Instance Data (DI)"=133, "Local Data (L)"=134, "Predecessor Local Data (VL)"=135] ("寄存器类型")
        n130 = case shown="1" w566 {
          tunnel: [u32 1 ("写入数据") u32 0 ("写入数据")] -> w561
          frame 0, Default {
          }
          frame 1 {
          }
        }
        "ST50 write" <- w561
        n131 = call "S7_Write.vi"("TCP"=w570, "寄存器类型"=w564, "DB #"=u16 7, "写入地址"=u32 2, "数据类型"=w562, "写入数据"=w561) -> ("TCP"=w569:refnum<k5>, "写入成功"=→"写入成功 5":bool, "error out"=w568:errorcluster)  [unwired: 7 in]
      }
      frame "错误" {
        n132 = call "S7_Close.vi"("TCP Connection Ref"=w578) -> ("error out"=w577:errorcluster)  [unwired: 10 in]
        n133 = call <vilib>:"Clear Errors.vi"("error in (no error)"=w577) -> ()  [unwired: 5 in, 2 out]
      }
    }
    n134 = local read "停止"() -> (w524:bool)
    n135 = case shown="假" w524 {
      tunnel: w526 -> [_ w536]
      tunnel: [FALSE TRUE] -> w525
      frame False {
      }
      frame True {
        n136 = call "S7_Close.vi"("TCP Connection Ref"=w536) -> ("error out"=w537:errorcluster)  [unwired: 10 in]
        n137 = call <vilib>:"Clear Errors.vi"("error in (no error)"=w537) -> ()  [unwired: 5 in, 2 out]
      }
    }
  }
  n138 = while {
    shift-right: [w584] -> _
    shift-left: 状态1."PLC通讯初始化" ("PLC状态") -> [w589]
    shift-right: [w586] -> _
    shift-left: errorcluster {"status"=FALSE, "code"=0, "source"=""} ("错误常量") -> [w590]
    shift-right: [w587] -> _
    shift-left: _ -> [w583]
    shift-right: [w579] -> _
    shift-left: u32 0 ("写入数据") -> [w580]
    stop <- w582 stop-if-true
    # "OP60"
    n139 = case shown="无错误" w590 {
      tunnel: w589 -> [w595 _]
      tunnel: [w595 状态1."错误" ("PLC状态")] -> w588
      frame No Error {
      }
      frame Error {
      }
    }
    n140 = Wait (ms)(milliseconds to wait=u32 100 ("等待时间（毫秒）")) -> ()  [unwired: 1 out]
    n141 = case shown="\"写DM\"" w588 {
      tunnel: [w601 w611 w626 refnum<k5> refnum ("TCP")] -> w587
      tunnel: [w598 w610 w625 errorcluster {"status"=FALSE, "code"=0, "source"=""} ("error out")] -> w586
      tunnel: w583 -> [_ w612 w627 w635]
      tunnel: [状态1."读DM" ("PLC状态") 状态1."写DM" ("PLC状态") 状态1."读DM" ("PLC状态") 状态1."PLC通讯初始化" ("PLC状态")] -> w584
      tunnel: w580 -> [w597 w606 w623 w630]
      tunnel: [w597 w606 w618 w630] -> w579
      frame "PLC通讯初始化", Default {
        w603 = u8 0 items=["S7-1200.200.200SMART"=0, "S7-300"=2, "S7-400"=3] ("PLC 系列")
        n142 = call "S7_Open.vi"("IP 地址"="192.168.0.60", "PLC 系列"=w603, "超时（MS）"=100) -> ("TCP"=w601:refnum<k5>, "error out"=w598:errorcluster)  [unwired: 10 in, 1 out]
        n143 = Unbundle By Name(w598) -> ("status"=→"ST60":bool)
      }
      frame "读DM" {
        w613 = u16 1 items=["byte", "word", "Dword"] ("数据类型")
        w615 = u8 132 items=["I/O (P)"=128, "Input (I)"=129, "Output (Q)"=130, "Bit Memory (M)"=131, "Data (DB)"=132, "Instance Data (DI)"=133, "Local Data (L)"=134, "Predecessor Local Data (VL)"=135] ("寄存器类型")
        n144 = call "S7_Read.vi"("TCP"=w612, "DB #"=u16 7, "读取长度"=u16 1, "寄存器类型"=w615, "起始地址"=u32 0, "数据类型"=w613) -> ("TCP"=w611:refnum<k5>, "数据"=→"ST60 read":u32[], "读取成功"=→"读取成功 13":bool, "error out"=w610:errorcluster)  [unwired: 6 in]
      }
      frame "写DM" {
        w619 = u16 1 items=["byte", "word", "Dword"] ("数据类型")
        w621 = u8 132 items=["I/O (P)"=128, "Input (I)"=129, "Output (Q)"=130, "Bit Memory (M)"=131, "Data (DB)"=132, "Instance Data (DI)"=133, "Local Data (L)"=134, "Predecessor Local Data (VL)"=135] ("寄存器类型")
        n145 = case shown="1" w623 {
          tunnel: [u32 1 ("写入数据") u32 0 ("写入数据")] -> w618
          frame 0, Default {
          }
          frame 1 {
          }
        }
        "ST60 write" <- w618
        n146 = call "S7_Write.vi"("TCP"=w627, "寄存器类型"=w621, "DB #"=u16 7, "写入地址"=u32 2, "数据类型"=w619, "写入数据"=w618) -> ("TCP"=w626:refnum<k5>, "写入成功"=→"写入成功 6":bool, "error out"=w625:errorcluster)  [unwired: 7 in]
      }
      frame "错误" {
        n147 = call "S7_Close.vi"("TCP Connection Ref"=w635) -> ("error out"=w634:errorcluster)  [unwired: 10 in]
        n148 = call <vilib>:"Clear Errors.vi"("error in (no error)"=w634) -> ()  [unwired: 5 in, 2 out]
      }
    }
    n149 = local read "停止"() -> (w581:bool)
    n150 = case shown="假" w581 {
      tunnel: w583 -> [_ w593]
      tunnel: [FALSE TRUE] -> w582
      frame False {
      }
      frame True {
        n151 = call "S7_Close.vi"("TCP Connection Ref"=w593) -> ("error out"=w594:errorcluster)  [unwired: 10 in]
        n152 = call <vilib>:"Clear Errors.vi"("error in (no error)"=w594) -> ()  [unwired: 5 in, 2 out]
      }
    }
  }
  n153 = while {
    shift-right: [w641] -> _
    shift-left: 状态1."PLC通讯初始化" ("PLC状态") -> [w646]
    shift-right: [w643] -> _
    shift-left: errorcluster {"status"=FALSE, "code"=0, "source"=""} ("错误常量") -> [w647]
    shift-right: [w644] -> _
    shift-left: _ -> [w640]
    shift-right: [w637] -> _
    shift-left: u32 0 ("写入数据") -> [w638]
    stop <- w639 stop-if-true
    # "OP100"
    n154 = case shown="无错误" w647 {
      tunnel: w646 -> [w652 _]
      tunnel: [w652 状态1."错误" ("PLC状态")] -> w645
      frame No Error {
      }
      frame Error {
      }
    }
    n155 = Wait (ms)(milliseconds to wait=u32 100 ("等待时间（毫秒）")) -> ()  [unwired: 1 out]
    n156 = case shown="\"读DM\"" w645 {
      tunnel: [w658 w668 w678 refnum<k5> refnum ("TCP")] -> w644
      tunnel: [w655 w667 w677 errorcluster {"status"=FALSE, "code"=0, "source"=""} ("error out")] -> w643
      tunnel: w640 -> [_ w669 w679 w699]
      tunnel: [状态1."读DM" ("PLC状态") 状态1."写DM" ("PLC状态") 状态1."读DM" ("PLC状态") 状态1."PLC通讯初始化" ("PLC状态")] -> w641
      tunnel: w638 -> [w654 w663 w675 w694]
      tunnel: [w654 w663 w674 w694] -> w637
      frame "PLC通讯初始化", Default {
        w660 = u8 0 items=["S7-1200.200.200SMART"=0, "S7-300"=2, "S7-400"=3] ("PLC 系列")
        n157 = call "S7_Open.vi"("IP 地址"="192.168.0.100", "PLC 系列"=w660, "超时（MS）"=100) -> ("TCP"=w658:refnum<k5>, "error out"=w655:errorcluster)  [unwired: 10 in, 1 out]
        n158 = Unbundle By Name(w655) -> ("status"=→"ST100":bool)
      }
      frame "读DM" {
        w670 = u16 0 items=["byte", "word", "Dword"] ("数据类型")
        w672 = u8 132 items=["I/O (P)"=128, "Input (I)"=129, "Output (Q)"=130, "Bit Memory (M)"=131, "Data (DB)"=132, "Instance Data (DI)"=133, "Local Data (L)"=134, "Predecessor Local Data (VL)"=135] ("寄存器类型")
        n159 = call "S7_Read.vi"("TCP"=w669, "DB #"=u16 4, "读取长度"=u16 1, "寄存器类型"=w672, "起始地址"=u32 0, "数据类型"=w670) -> ("TCP"=w668:refnum<k5>, "数据"=→"ST100 read":u32[], "读取成功"=→"读取成功 4":bool, "error out"=w667:errorcluster)  [unwired: 6 in]
      }
      frame "写DM" {
        n160 = disable-structure shown="启用" {
          disable-tunnel: w679 -> [w688 w692]
          disable-tunnel: [w687 w692] -> w678
          disable-tunnel: [w686 errorcluster {"status"=FALSE, "code"=0, "source"=""} ("error out")] -> w677
          disable-tunnel: w675 -> [w685 w693]
          disable-tunnel: [w680 w693] -> w674
          frame Disabled {
            w681 = u16 1 items=["byte", "word", "Dword"] ("数据类型")
            w683 = u8 132 items=["I/O (P)"=128, "Input (I)"=129, "Output (Q)"=130, "Bit Memory (M)"=131, "Data (DB)"=132, "Instance Data (DI)"=133, "Local Data (L)"=134, "Predecessor Local Data (VL)"=135] ("寄存器类型")
            n161 = case shown="1" w685 {
              tunnel: [u32 1 ("写入数据") u32 0 ("写入数据")] -> w680
              frame 0, Default {
              }
              frame 1 {
              }
            }
            "ST100 write" <- w680
            n162 = call "S7_Write.vi"("TCP"=w688, "寄存器类型"=w683, "DB #"=u16 7, "写入地址"=u32 2, "数据类型"=w681, "写入数据"=w680) -> ("TCP"=w687:refnum<k5>, "error out"=w686:errorcluster)  [unwired: 7 in, 1 out]
          }
          frame Enabled {
          }
        }
      }
      frame "错误" {
        n163 = call "S7_Close.vi"("TCP Connection Ref"=w699) -> ("error out"=w698:errorcluster)  [unwired: 10 in]
        n164 = call <vilib>:"Clear Errors.vi"("error in (no error)"=w698) -> ()  [unwired: 5 in, 2 out]
      }
    }
    n165 = local read "停止"() -> (w636:bool)
    n166 = case shown="假" w636 {
      tunnel: w640 -> [_ w650]
      tunnel: [FALSE TRUE] -> w639
      frame False {
      }
      frame True {
        n167 = call "S7_Close.vi"("TCP Connection Ref"=w650) -> ("error out"=w651:errorcluster)  [unwired: 10 in]
        n168 = call <vilib>:"Clear Errors.vi"("error in (no error)"=w651) -> ()  [unwired: 5 in, 2 out]
      }
    }
  }
  n169 = while {
    shift-right: [w705] -> _
    shift-left: 状态1."PLC通讯初始化" ("PLC状态") -> [w710]
    shift-right: [w707] -> _
    shift-left: errorcluster {"status"=FALSE, "code"=0, "source"=""} ("错误常量") -> [w711]
    shift-right: [w708] -> _
    shift-left: _ -> [w704]
    shift-right: [w701] -> _
    shift-left: u32 0 ("写入数据") -> [w702]
    stop <- w703 stop-if-true
    # "OP110"
    n170 = case shown="无错误" w711 {
      tunnel: w710 -> [w716 _]
      tunnel: [w716 状态1."错误" ("PLC状态")] -> w709
      frame No Error {
      }
      frame Error {
      }
    }
    n171 = Wait (ms)(milliseconds to wait=u32 100 ("等待时间（毫秒）")) -> ()  [unwired: 1 out]
    n172 = case shown="\"读DM\"" w709 {
      tunnel: [w722 w732 w742 refnum<k5> refnum ("TCP")] -> w708
      tunnel: [w719 w731 w741 errorcluster {"status"=FALSE, "code"=0, "source"=""} ("error out")] -> w707
      tunnel: w704 -> [_ w733 w743 w763]
      tunnel: [状态1."读DM" ("PLC状态") 状态1."写DM" ("PLC状态") 状态1."读DM" ("PLC状态") 状态1."PLC通讯初始化" ("PLC状态")] -> w705
      tunnel: w702 -> [w718 w727 w739 w758]
      tunnel: [w718 w727 w738 w758] -> w701
      frame "PLC通讯初始化", Default {
        w724 = u8 0 items=["S7-1200.200.200SMART"=0, "S7-300"=2, "S7-400"=3] ("PLC 系列")
        n173 = call "S7_Open.vi"("IP 地址"="192.168.0.110", "PLC 系列"=w724, "超时（MS）"=100) -> ("TCP"=w722:refnum<k5>, "error out"=w719:errorcluster)  [unwired: 10 in, 1 out]
        n174 = Unbundle By Name(w719) -> ("status"=→"ST110":bool)
      }
      frame "读DM" {
        w734 = u16 0 items=["byte", "word", "Dword"] ("数据类型")
        w736 = u8 132 items=["I/O (P)"=128, "Input (I)"=129, "Output (Q)"=130, "Bit Memory (M)"=131, "Data (DB)"=132, "Instance Data (DI)"=133, "Local Data (L)"=134, "Predecessor Local Data (VL)"=135] ("寄存器类型")
        n175 = call "S7_Read.vi"("TCP"=w733, "DB #"=u16 5, "读取长度"=u16 1, "寄存器类型"=w736, "起始地址"=u32 0, "数据类型"=w734) -> ("TCP"=w732:refnum<k5>, "数据"=→"ST110 read":u32[], "读取成功"=→"读取成功 5":bool, "error out"=w731:errorcluster)  [unwired: 6 in]
      }
      frame "写DM" {
        n176 = disable-structure shown="启用" {
          disable-tunnel: w743 -> [w752 w756]
          disable-tunnel: [w751 w756] -> w742
          disable-tunnel: [w750 errorcluster {"status"=FALSE, "code"=0, "source"=""} ("error out")] -> w741
          disable-tunnel: w739 -> [w749 w757]
          disable-tunnel: [w744 w757] -> w738
          frame Disabled {
            w745 = u16 1 items=["byte", "word", "Dword"] ("数据类型")
            w747 = u8 132 items=["I/O (P)"=128, "Input (I)"=129, "Output (Q)"=130, "Bit Memory (M)"=131, "Data (DB)"=132, "Instance Data (DI)"=133, "Local Data (L)"=134, "Predecessor Local Data (VL)"=135] ("寄存器类型")
            n177 = case shown="1" w749 {
              tunnel: [u32 1 ("写入数据") u32 0 ("写入数据")] -> w744
              frame 0, Default {
              }
              frame 1 {
              }
            }
            "ST110 write" <- w744
            n178 = call "S7_Write.vi"("TCP"=w752, "寄存器类型"=w747, "DB #"=u16 7, "写入地址"=u32 2, "数据类型"=w745, "写入数据"=w744) -> ("TCP"=w751:refnum<k5>, "error out"=w750:errorcluster)  [unwired: 7 in, 1 out]
          }
          frame Enabled {
          }
        }
      }
      frame "错误" {
        n179 = call "S7_Close.vi"("TCP Connection Ref"=w763) -> ("error out"=w762:errorcluster)  [unwired: 10 in]
        n180 = call <vilib>:"Clear Errors.vi"("error in (no error)"=w762) -> ()  [unwired: 5 in, 2 out]
      }
    }
    n181 = local read "停止"() -> (w700:bool)
    n182 = case shown="假" w700 {
      tunnel: w704 -> [_ w714]
      tunnel: [FALSE TRUE] -> w703
      frame False {
      }
      frame True {
        n183 = call "S7_Close.vi"("TCP Connection Ref"=w714) -> ("error out"=w715:errorcluster)  [unwired: 10 in]
        n184 = call <vilib>:"Clear Errors.vi"("error in (no error)"=w715) -> ()  [unwired: 5 in, 2 out]
      }
    }
  }
  n185 = while {
    shift-right: [w769] -> _
    shift-left: 状态1."PLC通讯初始化" ("PLC状态") -> [w774]
    shift-right: [w771] -> _
    shift-left: errorcluster {"status"=FALSE, "code"=0, "source"=""} ("错误常量") -> [w775]
    shift-right: [w772] -> _
    shift-left: _ -> [w768]
    shift-right: [w765] -> _
    shift-left: u32 0 ("写入数据") -> [w766]
    stop <- w767 stop-if-true
    # "OP120"
    n186 = case shown="无错误" w775 {
      tunnel: w774 -> [w780 _]
      tunnel: [w780 状态1."错误" ("PLC状态")] -> w773
      frame No Error {
      }
      frame Error {
      }
    }
    n187 = Wait (ms)(milliseconds to wait=u32 100 ("等待时间（毫秒）")) -> ()  [unwired: 1 out]
    n188 = case shown="\"读DM\"" w773 {
      tunnel: [w786 w796 w806 refnum<k5> refnum ("TCP")] -> w772
      tunnel: [w783 w795 w805 errorcluster {"status"=FALSE, "code"=0, "source"=""} ("error out")] -> w771
      tunnel: w768 -> [_ w797 w807 w827]
      tunnel: [状态1."读DM" ("PLC状态") 状态1."写DM" ("PLC状态") 状态1."读DM" ("PLC状态") 状态1."PLC通讯初始化" ("PLC状态")] -> w769
      tunnel: w766 -> [w782 w791 w803 w822]
      tunnel: [w782 w791 w802 w822] -> w765
      frame "PLC通讯初始化", Default {
        w788 = u8 0 items=["S7-1200.200.200SMART"=0, "S7-300"=2, "S7-400"=3] ("PLC 系列")
        n189 = call "S7_Open.vi"("IP 地址"="192.168.0.120", "PLC 系列"=w788, "超时（MS）"=100) -> ("TCP"=w786:refnum<k5>, "error out"=w783:errorcluster)  [unwired: 10 in, 1 out]
        n190 = Unbundle By Name(w783) -> ("status"=→"ST120":bool)
      }
      frame "读DM" {
        w798 = u16 0 items=["byte", "word", "Dword"] ("数据类型")
        w800 = u8 132 items=["I/O (P)"=128, "Input (I)"=129, "Output (Q)"=130, "Bit Memory (M)"=131, "Data (DB)"=132, "Instance Data (DI)"=133, "Local Data (L)"=134, "Predecessor Local Data (VL)"=135] ("寄存器类型")
        n191 = call "S7_Read.vi"("TCP"=w797, "DB #"=u16 1, "读取长度"=u16 1, "寄存器类型"=w800, "起始地址"=u32 0, "数据类型"=w798) -> ("TCP"=w796:refnum<k5>, "数据"=→"ST120 read":u32[], "读取成功"=→"读取成功 6":bool, "error out"=w795:errorcluster)  [unwired: 6 in]
      }
      frame "写DM" {
        n192 = disable-structure shown="启用" {
          disable-tunnel: w807 -> [w816 w820]
          disable-tunnel: [w815 w820] -> w806
          disable-tunnel: [w814 errorcluster {"status"=FALSE, "code"=0, "source"=""} ("error out")] -> w805
          disable-tunnel: w803 -> [w813 w821]
          disable-tunnel: [w808 w821] -> w802
          frame Disabled {
            w809 = u16 1 items=["byte", "word", "Dword"] ("数据类型")
            w811 = u8 132 items=["I/O (P)"=128, "Input (I)"=129, "Output (Q)"=130, "Bit Memory (M)"=131, "Data (DB)"=132, "Instance Data (DI)"=133, "Local Data (L)"=134, "Predecessor Local Data (VL)"=135] ("寄存器类型")
            n193 = case shown="1" w813 {
              tunnel: [u32 1 ("写入数据") u32 0 ("写入数据")] -> w808
              frame 0, Default {
              }
              frame 1 {
              }
            }
            "ST120 write" <- w808
            n194 = call "S7_Write.vi"("TCP"=w816, "寄存器类型"=w811, "DB #"=u16 7, "写入地址"=u32 2, "数据类型"=w809, "写入数据"=w808) -> ("TCP"=w815:refnum<k5>, "error out"=w814:errorcluster)  [unwired: 7 in, 1 out]
          }
          frame Enabled {
          }
        }
      }
      frame "错误" {
        n195 = call "S7_Close.vi"("TCP Connection Ref"=w827) -> ("error out"=w826:errorcluster)  [unwired: 10 in]
        n196 = call <vilib>:"Clear Errors.vi"("error in (no error)"=w826) -> ()  [unwired: 5 in, 2 out]
      }
    }
    n197 = local read "停止"() -> (w764:bool)
    n198 = case shown="假" w764 {
      tunnel: w768 -> [_ w778]
      tunnel: [FALSE TRUE] -> w767
      frame False {
      }
      frame True {
        n199 = call "S7_Close.vi"("TCP Connection Ref"=w778) -> ("error out"=w779:errorcluster)  [unwired: 10 in]
        n200 = call <vilib>:"Clear Errors.vi"("error in (no error)"=w779) -> ()  [unwired: 5 in, 2 out]
      }
    }
  }
  n201 = while {
    shift-right: [w833] -> _
    shift-left: 状态1."PLC通讯初始化" ("PLC状态") -> [w838]
    shift-right: [w835] -> _
    shift-left: errorcluster {"status"=FALSE, "code"=0, "source"=""} ("错误常量") -> [w839]
    shift-right: [w836] -> _
    shift-left: _ -> [w832]
    shift-right: [w829] -> _
    shift-left: u32 0 ("写入数据") -> [w830]
    stop <- w831 stop-if-true
    # "OP130"
    n202 = case shown="无错误" w839 {
      tunnel: w838 -> [w844 _]
      tunnel: [w844 状态1."错误" ("PLC状态")] -> w837
      frame No Error {
      }
      frame Error {
      }
    }
    n203 = Wait (ms)(milliseconds to wait=u32 100 ("等待时间（毫秒）")) -> ()  [unwired: 1 out]
    n204 = case shown="\"读DM\"" w837 {
      tunnel: [w850 w860 w870 refnum<k5> refnum ("TCP")] -> w836
      tunnel: [w847 w859 w869 errorcluster {"status"=FALSE, "code"=0, "source"=""} ("error out")] -> w835
      tunnel: w832 -> [_ w861 w871 w891]
      tunnel: [状态1."读DM" ("PLC状态") 状态1."写DM" ("PLC状态") 状态1."读DM" ("PLC状态") 状态1."PLC通讯初始化" ("PLC状态")] -> w833
      tunnel: w830 -> [w846 w855 w867 w886]
      tunnel: [w846 w855 w866 w886] -> w829
      frame "PLC通讯初始化", Default {
        w852 = u8 0 items=["S7-1200.200.200SMART"=0, "S7-300"=2, "S7-400"=3] ("PLC 系列")
        n205 = call "S7_Open.vi"("IP 地址"="192.168.0.130", "PLC 系列"=w852, "超时（MS）"=100) -> ("TCP"=w850:refnum<k5>, "error out"=w847:errorcluster)  [unwired: 10 in, 1 out]
        n206 = Unbundle By Name(w847) -> ("status"=→"ST130":bool)
      }
      frame "读DM" {
        w862 = u16 0 items=["byte", "word", "Dword"] ("数据类型")
        w864 = u8 132 items=["I/O (P)"=128, "Input (I)"=129, "Output (Q)"=130, "Bit Memory (M)"=131, "Data (DB)"=132, "Instance Data (DI)"=133, "Local Data (L)"=134, "Predecessor Local Data (VL)"=135] ("寄存器类型")
        n207 = call "S7_Read.vi"("TCP"=w861, "DB #"=u16 1, "读取长度"=u16 1, "寄存器类型"=w864, "起始地址"=u32 0, "数据类型"=w862) -> ("TCP"=w860:refnum<k5>, "数据"=→"ST130 read":u32[], "读取成功"=→"读取成功 7":bool, "error out"=w859:errorcluster)  [unwired: 6 in]
      }
      frame "写DM" {
        n208 = disable-structure shown="启用" {
          disable-tunnel: w871 -> [w880 w884]
          disable-tunnel: [w879 w884] -> w870
          disable-tunnel: [w878 errorcluster {"status"=FALSE, "code"=0, "source"=""} ("error out")] -> w869
          disable-tunnel: w867 -> [w877 w885]
          disable-tunnel: [w872 w885] -> w866
          frame Disabled {
            w873 = u16 1 items=["byte", "word", "Dword"] ("数据类型")
            w875 = u8 132 items=["I/O (P)"=128, "Input (I)"=129, "Output (Q)"=130, "Bit Memory (M)"=131, "Data (DB)"=132, "Instance Data (DI)"=133, "Local Data (L)"=134, "Predecessor Local Data (VL)"=135] ("寄存器类型")
            n209 = case shown="1" w877 {
              tunnel: [u32 1 ("写入数据") u32 0 ("写入数据")] -> w872
              frame 0, Default {
              }
              frame 1 {
              }
            }
            "ST130 write" <- w872
            n210 = call "S7_Write.vi"("TCP"=w880, "寄存器类型"=w875, "DB #"=u16 7, "写入地址"=u32 2, "数据类型"=w873, "写入数据"=w872) -> ("TCP"=w879:refnum<k5>, "error out"=w878:errorcluster)  [unwired: 7 in, 1 out]
          }
          frame Enabled {
          }
        }
      }
      frame "错误" {
        n211 = call "S7_Close.vi"("TCP Connection Ref"=w891) -> ("error out"=w890:errorcluster)  [unwired: 10 in]
        n212 = call <vilib>:"Clear Errors.vi"("error in (no error)"=w890) -> ()  [unwired: 5 in, 2 out]
      }
    }
    n213 = local read "停止"() -> (w828:bool)
    n214 = case shown="假" w828 {
      tunnel: w832 -> [_ w842]
      tunnel: [FALSE TRUE] -> w831
      frame False {
      }
      frame True {
        n215 = call "S7_Close.vi"("TCP Connection Ref"=w842) -> ("error out"=w843:errorcluster)  [unwired: 10 in]
        n216 = call <vilib>:"Clear Errors.vi"("error in (no error)"=w843) -> ()  [unwired: 5 in, 2 out]
      }
    }
  }
  n217 = while {
    shift-right: [w897] -> _
    shift-left: 状态1."PLC通讯初始化" ("PLC状态") -> [w902]
    shift-right: [w899] -> _
    shift-left: errorcluster {"status"=FALSE, "code"=0, "source"=""} ("错误常量") -> [w903]
    shift-right: [w900] -> _
    shift-left: _ -> [w896]
    shift-right: [w893] -> _
    shift-left: u32 0 ("写入数据") -> [w894]
    stop <- w895 stop-if-true
    # "OP140"
    n218 = case shown="无错误" w903 {
      tunnel: w902 -> [w908 _]
      tunnel: [w908 状态1."错误" ("PLC状态")] -> w901
      frame No Error {
      }
      frame Error {
      }
    }
    n219 = Wait (ms)(milliseconds to wait=u32 100 ("等待时间（毫秒）")) -> ()  [unwired: 1 out]
    n220 = case shown="\"错误\"" w901 {
      tunnel: [w914 w924 w934 refnum<k5> refnum ("TCP")] -> w900
      tunnel: [w911 w923 w933 errorcluster {"status"=FALSE, "code"=0, "source"=""} ("error out")] -> w899
      tunnel: w896 -> [_ w925 w935 w955]
      tunnel: [状态1."读DM" ("PLC状态") 状态1."写DM" ("PLC状态") 状态1."读DM" ("PLC状态") 状态1."PLC通讯初始化" ("PLC状态")] -> w897
      tunnel: w894 -> [w910 w919 w931 w950]
      tunnel: [w910 w919 w930 w950] -> w893
      frame "PLC通讯初始化", Default {
        w916 = u8 0 items=["S7-1200.200.200SMART"=0, "S7-300"=2, "S7-400"=3] ("PLC 系列")
        n221 = call "S7_Open.vi"("IP 地址"="192.168.0.140", "PLC 系列"=w916, "超时（MS）"=100) -> ("TCP"=w914:refnum<k5>, "error out"=w911:errorcluster)  [unwired: 10 in, 1 out]
        n222 = Unbundle By Name(w911) -> ("status"=→"ST140":bool)
      }
      frame "读DM" {
        w926 = u16 0 items=["byte", "word", "Dword"] ("数据类型")
        w928 = u8 132 items=["I/O (P)"=128, "Input (I)"=129, "Output (Q)"=130, "Bit Memory (M)"=131, "Data (DB)"=132, "Instance Data (DI)"=133, "Local Data (L)"=134, "Predecessor Local Data (VL)"=135] ("寄存器类型")
        n223 = call "S7_Read.vi"("TCP"=w925, "DB #"=u16 1, "读取长度"=u16 1, "寄存器类型"=w928, "起始地址"=u32 0, "数据类型"=w926) -> ("TCP"=w924:refnum<k5>, "数据"=→"ST140 read":u32[], "读取成功"=→"读取成功 8":bool, "error out"=w923:errorcluster)  [unwired: 6 in]
      }
      frame "写DM" {
        n224 = disable-structure shown="启用" {
          disable-tunnel: w935 -> [w944 w948]
          disable-tunnel: [w943 w948] -> w934
          disable-tunnel: [w942 errorcluster {"status"=FALSE, "code"=0, "source"=""} ("error out")] -> w933
          disable-tunnel: w931 -> [w941 w949]
          disable-tunnel: [w936 w949] -> w930
          frame Disabled {
            w937 = u16 1 items=["byte", "word", "Dword"] ("数据类型")
            w939 = u8 132 items=["I/O (P)"=128, "Input (I)"=129, "Output (Q)"=130, "Bit Memory (M)"=131, "Data (DB)"=132, "Instance Data (DI)"=133, "Local Data (L)"=134, "Predecessor Local Data (VL)"=135] ("寄存器类型")
            n225 = case shown="1" w941 {
              tunnel: [u32 1 ("写入数据") u32 0 ("写入数据")] -> w936
              frame 0, Default {
              }
              frame 1 {
              }
            }
            "ST140 write" <- w936
            n226 = call "S7_Write.vi"("TCP"=w944, "寄存器类型"=w939, "DB #"=u16 7, "写入地址"=u32 2, "数据类型"=w937, "写入数据"=w936) -> ("TCP"=w943:refnum<k5>, "error out"=w942:errorcluster)  [unwired: 7 in, 1 out]
          }
          frame Enabled {
          }
        }
      }
      frame "错误" {
        n227 = call "S7_Close.vi"("TCP Connection Ref"=w955) -> ("error out"=w954:errorcluster)  [unwired: 10 in]
        n228 = call <vilib>:"Clear Errors.vi"("error in (no error)"=w954) -> ()  [unwired: 5 in, 2 out]
      }
    }
    n229 = local read "停止"() -> (w892:bool)
    n230 = case shown="假" w892 {
      tunnel: w896 -> [_ w906]
      tunnel: [FALSE TRUE] -> w895
      frame False {
      }
      frame True {
        n231 = call "S7_Close.vi"("TCP Connection Ref"=w906) -> ("error out"=w907:errorcluster)  [unwired: 10 in]
        n232 = call <vilib>:"Clear Errors.vi"("error in (no error)"=w907) -> ()  [unwired: 5 in, 2 out]
      }
    }
  }
